vi "Advance Channel.vi"(8 "error in (no error)":errorcluster, 11 "Channel Scanner Driver in":refnum<class "Channel Scanner Driver.lvclass">) -> (0 "error out":errorcluster, 1 "Next channel":i32, 2 "Current channel":i32, 3 "Channel Scanner Driver out":refnum<class "Channel Scanner Driver.lvclass">)   [LabVIEW 2016, in "Channel Scanner Driver.lvclass"]
uses:
  Channel Scanner Driver.lvclass
  Channel Scanner Driver.lvclass/Channel Scanner Driver.ctl
  Read Next channel idx.vi
  Read Scan Channels.vi
  Write Next channel idx.vi
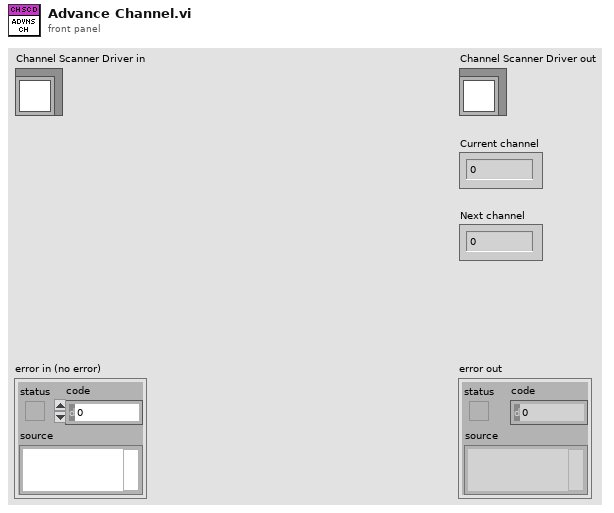
[diagram p1: front panel]
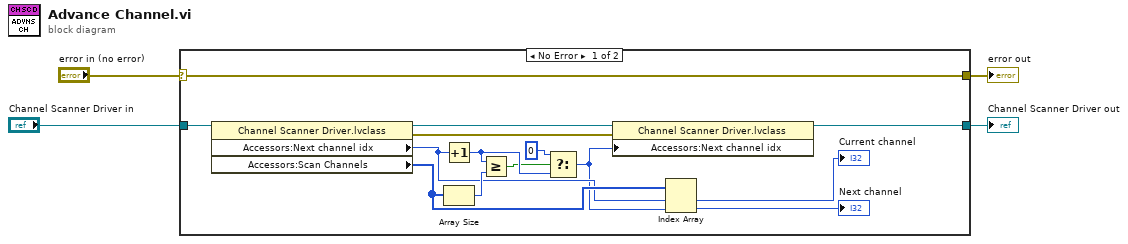
[diagram p0: block diagram]
diagram:
  n1 = case shown="No Error" "error in (no error)" {
    selector: "error in (no error)" -> [w17 w20]
    tunnel: [w17 w20] -> w3
    tunnel: [w11 w19] -> w1
    tunnel: "Channel Scanner Driver in" -> [w18 w19]
    frame No Error {
      n2 = property class="Channel Scanner Driver.lvclass"(reference=w18) -> (reference out=w16:refnum<class "Channel Scanner Driver.lvclass">, error out=w10:errorcluster, "Accessors:Next channel idx"=w8:i32, "Accessors:Scan Channels"=w9:i32[])  [unwired: 1 in]
      n3 = Increment(x=w8) -> (x+1=w15:i32)
      n4 = Array Size(array=w9) -> (size(s)=w12:i32)
      n5 = Greater Or Equal?(x=w15, y=w12) -> (x >= y?=w13:bool)
      n6 = Select(t=0, s=w13, f=w15) -> (s? t:f=w7:i32)
      n7 = property class="Channel Scanner Driver.lvclass"(reference=w16, error in=w10, "Accessors:Next channel idx"=w7) -> (reference out=w11:refnum<class "Channel Scanner Driver.lvclass">)  [unwired: 1 out]
      n8 = Index Array(array=w9, index #1=w8, index #2=w7) -> (element #1=→"Current channel":i32, element #2=→"Next channel":i32)
    }
    frame Error {
    }
  }
  "error out" <- w3
  "Channel Scanner Driver out" <- w1
